vi "Read Lossless.vi"(0 "Depth (Unlimited)":i32=-1, 1 "Timeout mS (-1)":i32=-1, 2 "FlexChannel":T2, 3 "Release (F)":bool) -> (5 "Timed Out?":bool, 7 "Element":T1, 8 "Closed?":bool)   [LabVIEW 2020, in "Flex.lvlib"]
doc: "Reads data losslessly from the channel just like a Queue. The <b>Depth</b> (Max Size) of the queue can be set to a specific value to be able to throttle the writer. Be aware that causing the writer to throttle will may affect the operation of parallel readers if they expect to run unimpeded.\n\nIn order to prevent leaking references, ensure that <b>Release</b> is set to true for the last call before code stops running. If <b>Closed?</b> has returned true then the loop can cleanly close down without setting <b>Release</b> for an iteration."
uses:
  Flex.lvlib
  ))Channel.ctl
  Element.ctl
  ChannelOp.ctl
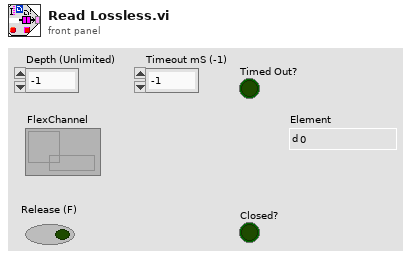
[diagram p1: front panel]
types:
  T1 = typedef "Flex.lvlib/Element.ctl" = dbl
  T2 = typedef "Flex.lvlib/))Channel.ctl" = refnum<queue>
  T3 = typedef "Flex.lvlib/ChannelOp.ctl" = enum16{"Get Refs", "Init", "Close", "Probe", "New Queue", "Remove Queue"}
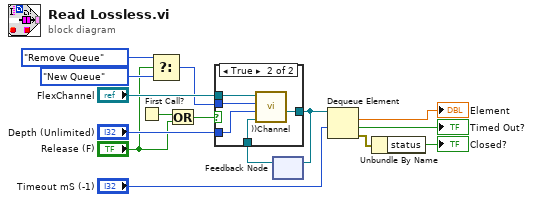
[diagram p0: block diagram]
diagram:
  n1 = First Call?() -> (First Call?: T/F=w3:bool)
  n2 = Select(t=ChannelOp."Remove Queue" ("channelOp"), s="Release (F)", f=ChannelOp."New Queue" ("channelOp")) -> (s? t:f=w4:T3)
  n3 = Or(x=w3, y="Release (F)") -> (x .or. y?=w2:bool)
  n4 = feedback #1() -> (w9:refnum<queue>)  [unwired: 1 in]
  n5 = case shown="True" w2 {
    tunnel: "FlexChannel" -> [_ w21]
    tunnel: w4 -> [_ w20]
    tunnel: w9 -> [w16 w17]
    tunnel: "Depth (Unlimited)" -> [_ w19]
    tunnel: [w16 w18] -> w8
    frame False {
    }
    frame True {
      n6 = call "))Channel.vi"("Remove Queue"=w17, "New Queue Depth"=w19, "channelOp"=w20, "channel in"=w21) -> ("New Queue"=w18:refnum<queue>)  [unwired: 4 in, 3 out]
    }
  }
  n7 = feedback-in #1(w8) -> ()
  n8 = Dequeue Element(queue=w8, timeout in ms (-1)="Timeout mS (-1)") -> (element=→"Element":T1, timed out?=→"Timed Out?":bool, error out=w7:errorcluster)  [unwired: 1 in, 1 out]
  n9 = Unbundle By Name(w7) -> ("status"=→"Closed?":bool)
